vi "test-traj-generate-8-way.vi"() -> ()   [LabVIEW 2019]
uses:
  <vilib>/Rock Robotics/WPI/ThirdParty/JAS_Junk/TrajLib/TRAJECTORY.ctl
  <vilib>/Rock Robotics/WPI/ThirdParty/JAS_Junk/TrajLib/TRAJ_STATE.ctl
  <vilib>/Rock Robotics/WPI/ThirdParty/JAS_Junk/TrajLib/POSE2D.ctl
  <vilib>/Rock Robotics/WPI/ThirdParty/JAS_Junk/TrajLib/TRANSLATION2D.ctl
  <vilib>/Rock Robotics/WPI/ThirdParty/JAS_Junk/TrajLib/ROTATION2D.ctl
  <vilib>/Rock Robotics/WPI/ThirdParty/JAS_Junk/TrajLib/UTIL_WAYPOINT.ctl
  <vilib>/Rock Robotics/WPI/ThirdParty/JAS_Junk/TrajLib/SPLINE.ctl
  <vilib>/Analysis/Matrix/Datatypes/RealMatrix.ctl
  <vilib>/Rock Robotics/WPI/ThirdParty/JAS_Junk/TrajLib/POSEwCURVATURE.ctl
  <vilib>/Rock Robotics/WPI/ThirdParty/JAS_Junk/TrajLib/TRAJ_CONFIG.ctl
  <vilib>/Rock Robotics/WPI/ThirdParty/JAS_Junk/TrajLib/TRAJ_CONSTRAINT_DIIF_DRIVE_KINEMATICS.ctl
  <vilib>/Rock Robotics/WPI/ThirdParty/JAS_Junk/TrajLib/DIFF_DRIVE_KINEMATICS.ctl
  <vilib>/Rock Robotics/WPI/ThirdParty/JAS_Junk/TrajLib/TRAJ_CONSTRAINT_CENTRIPETAL_ACCEL.ctl
  <vilib>/Rock Robotics/WPI/ThirdParty/JAS_Junk/TrajLib/TRAJ_CONSTRAINT_SWERVE_DRIVE_KINEMATICS.ctl
  <vilib>/Rock Robotics/WPI/ThirdParty/JAS_Junk/TrajLib/SWERVE_DRIVE_KINEMATICS.ctl
  <vilib>/Rock Robotics/WPI/ThirdParty/JAS_Junk/TrajLib/TRAJ_CONSTRAINT_DIIF_DRIVE_VOLTAGE.ctl
  <vilib>/Rock Robotics/WPI/ThirdParty/JAS_Junk/TrajLib/SIMPLE_MOTOR_FF.ctl
  <vilib>/Rock Robotics/WPI/ThirdParty/JAS_Junk/TrajLib/TRAJ_CONSTRAINT_MECA_DRIVE_KINEMATICS.ctl
  <vilib>/Rock Robotics/WPI/ThirdParty/JAS_Junk/TrajLib/MECA_DRIVE_KINEMATICS.ctl
  <vilib>/Rock Robotics/WPI/ThirdParty/JAS_Junk/TrajLib/UTIL_WEIGHTED_WAYPOINT.ctl
  <vilib>/Rock Robotics/SystemInterfaces/NetworkCommunication/NetComm_UsageReport_report.vi
  <vilib>/Rock Robotics/WPI/ThirdParty/JAS_Junk/TrajLib/DiffDriveKinematicsConstraint_New.vi
  <vilib>/Rock Robotics/WPI/ThirdParty/JAS_Junk/TrajLib/CentripetalAccelConstraint_New.vi
  <vilib>/Rock Robotics/WPI/ThirdParty/JAS_Junk/TrajLib/Rotation_CreateAngle.vi
  <vilib>/Rock Robotics/WPI/ThirdParty/JAS_Junk/TrajLib/Translation_Create.vi
  <vilib>/Rock Robotics/WPI/ThirdParty/JAS_Junk/TrajLib/Util_LibraryGlobals.vi
  <vilib>/Rock Robotics/WPI/ThirdParty/JAS_Junk/TrajLib/Trajectory_Library.lvlib
  <vilib>/Analysis/Matrix/NI_Matrix.lvlib
panel:
  in  "Tab Control":T1(tab)
  in  "Interior WAYPOINTS":T2[](array[typedef])=[{"X"=1.5, "Y"=1.5}, {"X"=0.0, "Y"=0.0}, {"X"=-1.5, "Y"=-1.5}, {"X"=-3.0, "Y"=0.0}, {"X"=-1.5, "Y"=1.5}, {"X"=0.0, "Y"=0.0}, {"X"=1.5, "Y"=-1.5}] {"Y" format="%14.3f"; "X" format="%14.3f"}
  in  "Initial_Position":T3={"X"=3.0, "Y"=0.0, "ANGLE"=1.571} {"ANGLE" format="%13.3f"; "Y" format="%13.3f"; "X" format="%13.3f"}
  in  "Ending_Position":T3={"X"=3.0, "Y"=0.0, "ANGLE"=1.571} {"ANGLE" format="%13.3f"; "Y" format="%13.3f"; "X" format="%13.3f"}
  out "splines":T4[](array[typedef])
  out "ArrayPoseWithCurvature":T6[](array[typedef]) {"POSE"."ROTATION"."SIN" format="%13.4f"; "POSE"."ROTATION"."COS" format="%13.4f"; "POSE"."ROTATION"."VALUE" format="%13.4f"; "POSE"."TRANSLATION"."Y" format="%14.3f"; "POSE"."TRANSLATION"."X" format="%14.3f"}
  out "PoseCSize":i32
  out "error out 2":errorcluster
  in  "MaxVelocity":dbl=2.0 format="%17.4f"
  in  "MaxAcceleration":dbl=1.3 format="%17.4f"
  in  "TrackWidth_Meters":dbl=0.66 format="%20.4f"
  in  "Max Cent Accel":dbl=1.0 format="%20.4f"
  out "outTRAJECTORY_CONFIG":T9={"MaxVelocity"=0.0, "Max Acceleration"=0.0, "StartVelocity"=0.0, "End Velocity"=0.0, "Reversed"=FALSE, "DiffDrKineConstntDefined"=FALSE, "CentAcellConstntDefined"=FALSE, "DiffDrVoltConstntDefined"=FALSE, "DIFF_DRIVE_KINE_CONSTRAINT"={"Max Speed (M/S)"=0.0, "DIFF_DRIVE_KINEMATICS"={"TrackWidth_Meters"=0.0}}, "CENTRIPETAL_ACCEL_CONSTRAINT"={"Max Cent Accel"=0.0}, "SwerveDrKineConstntDefined"=FALSE, "SWERVE_DRIVE_KINE_CONSTRAINT"={"Max Speed (M/S)"=0.0, "SwerveKinematics"={"NumModules"=0, "InverseKinematics"=[], "ForwardKinematics"=[], "Modules"=[], "PrevCoR"={"X"=0.0, "Y"=0.0}}}, "DIFF_DRIVE_VOLTAGE_CONSTRAINT"={"Max Voltage"=0.0, "DIFF_DRIVE_KINEMATICS"={"TrackWidth_Meters"=0.0}, "SIMPLE_MOTOR_FF"={"Ks"=0.0, "Kv"=0.0, "Ka"=0.0}}, "MECANUM_DRIVE_KINE_CONSTRAINT"={"Max Speed (M/S)"=0.0, "MECA_DRIVE_KINEMATICS"={"FrontLeft"={"X"=0.0, "Y"=0.0}, "FrontRight"={"X"=0.0, "Y"=0.0}, "RearLeft"={"X"=0.0, "Y"=0.0}, "RearRight"={"X"=0.0, "Y"=0.0}, "InverseKinematics"=[[0.0, 1.0, -1.0, 0.0], [0.0, 1.0, 1.0, 0.0], [0.0, 1.0, 1.0, 0.0], [0.0, 1.0, -1.0, 0.0]], "ForwardKinematics"=[[0.0, 1.0, -1.0, 0.0], [0.0, 1.0, 1.0, 0.0], [0.0, 1.0, 1.0, 0.0], [0.0, 1.0, -1.0, 0.0]], "PrevCoR"={"X"=0.0, "Y"=0.0}}}, "MecanumDrKineConstntDefined"=FALSE} {"MECANUM_DRIVE_KINE_CONSTRAINT"."MECA_DRIVE_KINEMATICS"."PrevCoR"."Y" format="%14.3f"; "MECANUM_DRIVE_KINE_CONSTRAINT"."MECA_DRIVE_KINEMATICS"."PrevCoR"."X" format="%14.3f"; "MECANUM_DRIVE_KINE_CONSTRAINT"."MECA_DRIVE_KINEMATICS"."RearRight"."Y" format="%14.3f"; "MECANUM_DRIVE_KINE_CONSTRAINT"."MECA_DRIVE_KINEMATICS"."RearRight"."X" format="%14.3f"; "MECANUM_DRIVE_KINE_CONSTRAINT"."MECA_DRIVE_KINEMATICS"."RearLeft"."Y" format="%14.3f"; "MECANUM_DRIVE_KINE_CONSTRAINT"."MECA_DRIVE_KINEMATICS"."RearLeft"."X" format="%14.3f"; "MECANUM_DRIVE_KINE_CONSTRAINT"."MECA_DRIVE_KINEMATICS"."FrontRight"."Y" format="%14.3f"; "MECANUM_DRIVE_KINE_CONSTRAINT"."MECA_DRIVE_KINEMATICS"."FrontRight"."X" format="%14.3f"; "MECANUM_DRIVE_KINE_CONSTRAINT"."MECA_DRIVE_KINEMATICS"."FrontLeft"."Y" format="%14.3f"; "MECANUM_DRIVE_KINE_CONSTRAINT"."MECA_DRIVE_KINEMATICS"."FrontLeft"."X" format="%14.3f"; "MECANUM_DRIVE_KINE_CONSTRAINT"."Max Speed (M/S)" format="%20.4f"; "DIFF_DRIVE_VOLTAGE_CONSTRAINT"."SIMPLE_MOTOR_FF"."Ka" format="%13.4f"; "DIFF_DRIVE_VOLTAGE_CONSTRAINT"."SIMPLE_MOTOR_FF"."Kv" format="%13.4f"; "DIFF_DRIVE_VOLTAGE_CONSTRAINT"."SIMPLE_MOTOR_FF"."Ks" format="%13.4f"; "DIFF_DRIVE_VOLTAGE_CONSTRAINT"."DIFF_DRIVE_KINEMATICS"."TrackWidth_Meters" format="%20.4f"; "DIFF_DRIVE_VOLTAGE_CONSTRAINT"."Max Voltage" format="%20.4f"; "SWERVE_DRIVE_KINE_CONSTRAINT"."SwerveKinematics"."PrevCoR"."Y" format="%14.3f"; "SWERVE_DRIVE_KINE_CONSTRAINT"."SwerveKinematics"."PrevCoR"."X" format="%14.3f"; "SWERVE_DRIVE_KINE_CONSTRAINT"."SwerveKinematics"."Modules"."Y" format="%14.3f"; "SWERVE_DRIVE_KINE_CONSTRAINT"."SwerveKinematics"."Modules"."X" format="%14.3f"; "SWERVE_DRIVE_KINE_CONSTRAINT"."Max Speed (M/S)" format="%20.4f"; "CENTRIPETAL_ACCEL_CONSTRAINT"."Max Cent Accel" format="%20.4f"; "DIFF_DRIVE_KINE_CONSTRAINT"."DIFF_DRIVE_KINEMATICS"."TrackWidth_Meters" format="%20.4f"; "DIFF_DRIVE_KINE_CONSTRAINT"."Max Speed (M/S)" format="%20.4f"; "End Velocity" format="%20.4f"; "StartVelocity" format="%20.4f"; "Max Acceleration" format="%20.4f"; "MaxVelocity" format="%20.4f"}
  out "TRAJECTORY":T19 {"States"."POSE"."ROTATION"."SIN" format="%13.4f"; "States"."POSE"."ROTATION"."COS" format="%13.4f"; "States"."POSE"."ROTATION"."VALUE" format="%13.4f"; "States"."POSE"."TRANSLATION"."Y" format="%14.3f"; "States"."POSE"."TRANSLATION"."X" format="%14.3f"; "TotalTImeSecs" format="%20.3f"}
  out "size(s)":i32
  out "error out":errorcluster
  out "read Traj":errorcluster
  out "readTRAJECTORY":T19 {"States"."POSE"."ROTATION"."SIN" format="%13.4f"; "States"."POSE"."ROTATION"."COS" format="%13.4f"; "States"."POSE"."ROTATION"."VALUE" format="%13.4f"; "States"."POSE"."TRANSLATION"."Y" format="%14.3f"; "States"."POSE"."TRANSLATION"."X" format="%14.3f"; "TotalTImeSecs" format="%20.3f"}
  out "size(s) 2":i32
  out "file write error":errorcluster
  out "appended path":path
  out "XY Graph":cluster{dbl[], dbl[]}(graph)
  out "Position":cluster{dbl[], dbl[]}(graph)
  out "Time":dbl
  in  "STEP":bool
  out "XY Graph 2":cluster{dbl[], dbl[]}(graph)
  out "TimeSeconds":dbl
  out "OutputTRAJ_STATE":T20={"TimeSeconds"=0.0, "Velocity"=0.0, "Acceleration"=0.0, "POSE"={"TRANSLATION"={"X"=0.0, "Y"=0.0}, "ROTATION"={"VALUE"=0.0, "COS"=1.0, "SIN"=0.0}}, "Curvature"=0.0} {"POSE"."ROTATION"."SIN" format="%13.4f"; "POSE"."ROTATION"."COS" format="%13.4f"; "POSE"."ROTATION"."VALUE" format="%13.4f"; "POSE"."TRANSLATION"."Y" format="%14.3f"; "POSE"."TRANSLATION"."X" format="%14.3f"}
  in  "CONT":bool
  out "Done":bool
  # "ARRAY OF OTHER\nCONSTRAINTS \nGOES HERE.."
  # "Single step\nthrough \ntrajectory"
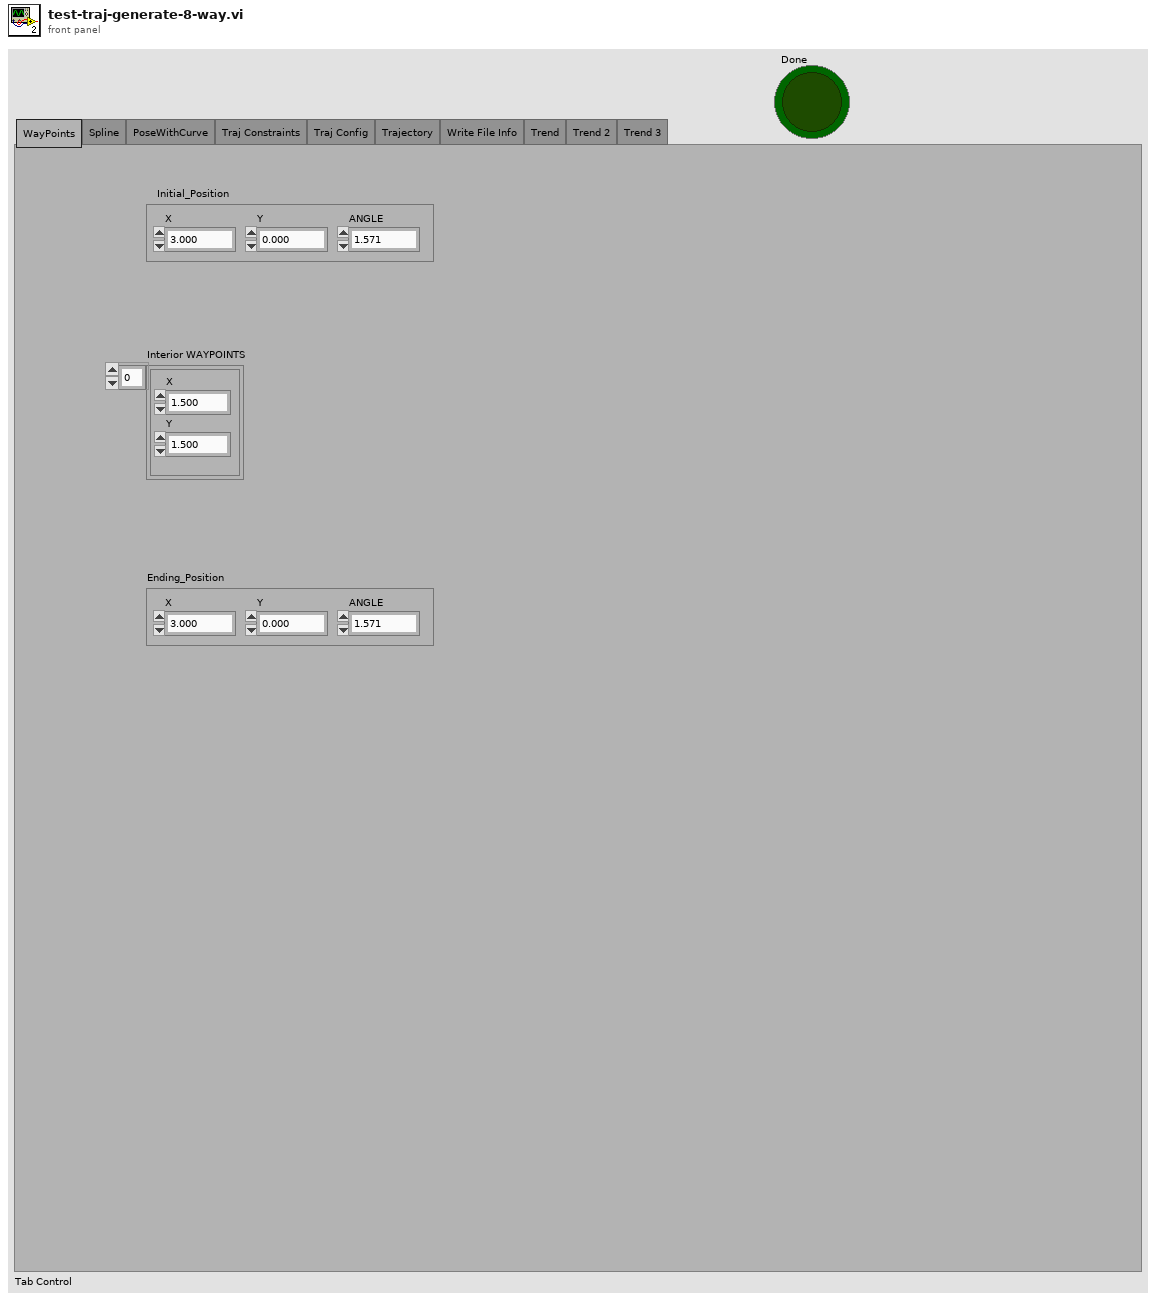
[diagram p1: front panel]
types:
  T1 = enum32{"WayPoints", "Spline", "PoseWithCurve", "Traj Constraints", "Traj Config", "Trajectory", "Write File Info", "Trend", "Trend 2", "Trend 3"}
  T2 = typedef "Trajectory_Library.lvlib/TRANSLATION2D.ctl" = cluster{"X":dbl, "Y":dbl}
  T3 = typedef "Trajectory_Library.lvlib/UTIL_WAYPOINT.ctl" = cluster{"X":dbl, "Y":dbl, "ANGLE":dbl}
  T4 = typedef "Trajectory_Library.lvlib/SPLINE.ctl" = cluster{"Degree":i32, "Coefficients":T5}
  T5 = typedef "NI_Matrix.lvlib/RealMatrix.ctl" = dbl[][]
  T6 = typedef "Trajectory_Library.lvlib/POSEwCURVATURE.ctl" = cluster{"CURVATURE":dbl, "POSE":T7}
  T7 = typedef "Trajectory_Library.lvlib/POSE2D.ctl" = cluster{"TRANSLATION":T2, "ROTATION":T8}
  T8 = typedef "Trajectory_Library.lvlib/ROTATION2D.ctl" = cluster{"VALUE":dbl, "COS":dbl, "SIN":dbl}
  T9 = typedef "Trajectory_Library.lvlib/TRAJ_CONFIG.ctl" = cluster{"MaxVelocity":dbl, "Max Acceleration":dbl, "StartVelocity":dbl, "End Velocity":dbl, "Reversed":bool, "DiffDrKineConstntDefined":bool, "CentAcellConstntDefined":bool, "DiffDrVoltConstntDefined":bool, "DIFF_DRIVE_KINE_CONSTRAINT":T10, "CENTRIPETAL_ACCEL_CONSTRAINT":T12, "SwerveDrKineConstntDefined":bool, "SWERVE_DRIVE_KINE_CONSTRAINT":T13, "DIFF_DRIVE_VOLTAGE_CONSTRAINT":T15, "MECANUM_DRIVE_KINE_CONSTRAINT":T17, "MecanumDrKineConstntDefined":bool}
  T10 = typedef "Trajectory_Library.lvlib/TRAJ_CONSTRAINT_DIIF_DRIVE_KINEMATICS.ctl" = cluster{"Max Speed (M/S)":dbl, "DIFF_DRIVE_KINEMATICS":T11}
  T11 = typedef "Trajectory_Library.lvlib/DIFF_DRIVE_KINEMATICS.ctl" = cluster{"TrackWidth_Meters":dbl}
  T12 = typedef "Trajectory_Library.lvlib/TRAJ_CONSTRAINT_CENTRIPETAL_ACCEL.ctl" = cluster{"Max Cent Accel":dbl}
  T13 = typedef "Trajectory_Library.lvlib/TRAJ_CONSTRAINT_SWERVE_DRIVE_KINEMATICS.ctl" = cluster{"Max Speed (M/S)":dbl, "SwerveKinematics":T14}
  T14 = typedef "Trajectory_Library.lvlib/SWERVE_DRIVE_KINEMATICS.ctl" = cluster{"NumModules":i32, "InverseKinematics":T5, "ForwardKinematics":T5, "Modules":T2[], "PrevCoR":T2}
  T15 = typedef "Trajectory_Library.lvlib/TRAJ_CONSTRAINT_DIIF_DRIVE_VOLTAGE.ctl" = cluster{"Max Voltage":dbl, "DIFF_DRIVE_KINEMATICS":T11, "SIMPLE_MOTOR_FF":T16}
  T16 = typedef "Trajectory_Library.lvlib/SIMPLE_MOTOR_FF.ctl" = cluster{"Ks":dbl, "Kv":dbl, "Ka":dbl}
  T17 = typedef "Trajectory_Library.lvlib/TRAJ_CONSTRAINT_MECA_DRIVE_KINEMATICS.ctl" = cluster{"Max Speed (M/S)":dbl, "MECA_DRIVE_KINEMATICS":T18}
  T18 = typedef "Trajectory_Library.lvlib/MECA_DRIVE_KINEMATICS.ctl" = cluster{"FrontLeft":T2, "FrontRight":T2, "RearLeft":T2, "RearRight":T2, "InverseKinematics":T5, "ForwardKinematics":T5, "PrevCoR":T2}
  T19 = typedef "Trajectory_Library.lvlib/TRAJECTORY.ctl" = cluster{"TotalTImeSecs":dbl, "States":T20[]}
  T20 = typedef "Trajectory_Library.lvlib/TRAJ_STATE.ctl" = cluster{"TimeSeconds":dbl, "Velocity":dbl, "Acceleration":dbl, "POSE":T7, "Curvature":dbl}
  T21 = typedef "Trajectory_Library.lvlib/UTIL_WEIGHTED_WAYPOINT.ctl" = cluster{"X":dbl, "Y":dbl, "ANGLE":dbl, "WEIGHT":dbl}
  T22 = typedef "Trajectory_Library.lvlib/SPLINE_CTRL_VECTOR.ctl" = cluster{"Xs":dbl[], "Ys":dbl[]}
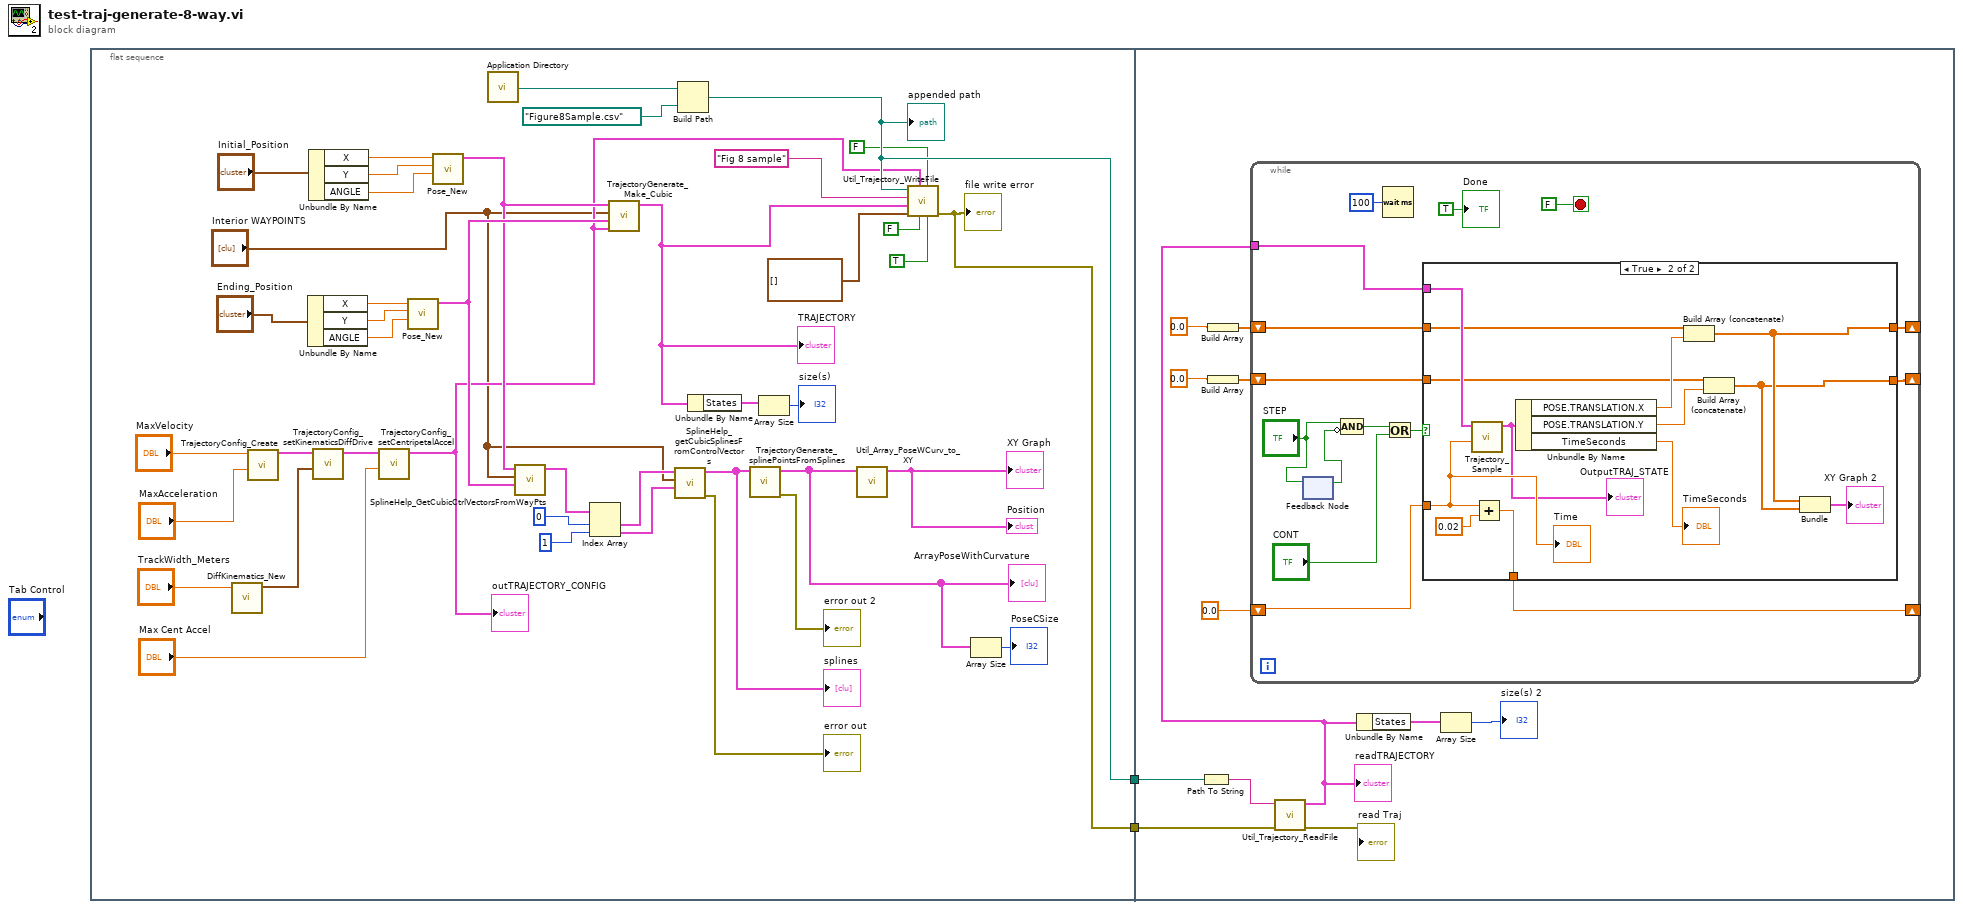
[diagram p0: block diagram]
diagram:
  n1 = flat-sequence {
    tunnel: [w11] -> w2
    tunnel: [w3] -> w1
    tunnel: w2 -> [w49]
    tunnel: w1 -> [w45]
    frame #0 {
      n2 = call <vilib>:"DiffKinematics_New.vi"("TrackWidth_Meters"="TrackWidth_Meters") -> ("DIFF_DRIVE_KINEMATICS"=w16:T11)  [unwired: 10 in]
      n3 = call <vilib>:"TrajectoryConfig_Create.vi"("MaxAcceleration"="MaxAcceleration", "MaxVelocity"="MaxVelocity") -> ("TRAJECTORY_CONFIG"=w18:T9)  [unwired: 9 in]
      n4 = Unbundle By Name("Ending_Position") -> ("X"=w40:dbl, "Y"=w39:dbl, "ANGLE"=w38:dbl)
      n5 = Unbundle By Name("Initial_Position") -> ("X"=w43:dbl, "Y"=w42:dbl, "ANGLE"=w41:dbl)
      n6 = call <vilib>:"TrajectoryConfig_setKinematicsDiffDrive.vi"("DIFF_DRIVE_KINEMATICS"=w16, "inTRAJECTORY_CONFIG"=w18) -> ("outTRAJECTORY_CONFIG"=w15:T9)  [unwired: 9 in]
      n7 = call <vilib>:"TrajectoryConfig_setCentripetalAccel.vi"("Max Cent Accel"="Max Cent Accel", "inTRAJECTORY_CONFIG"=w15) -> ("outTRAJECTORY_CONFIG"=w10:T9)  [unwired: 9 in]
      "outTRAJECTORY_CONFIG" <- w10
      n8 = call <vilib>:"Pose_New.vi"("Heading"=w38, "Y"=w39, "X"=w40) -> ("out POSe"=w36:T7)  [unwired: 8 in]
      n9 = call <vilib>:"Pose_New.vi"("Heading"=w41, "Y"=w42, "X"=w43) -> ("out POSe"=w35:T7)  [unwired: 8 in]
      n10 = call <vilib>:"Application Directory.vi"() -> ("Application Directory"=w12:path)
      n11 = call <vilib>:"SplineHelp_GetCubicCtrlVectorsFromWayPts.vi"("Enging POSE"=w36, "Interior WAYPOINTS"="Interior WAYPOINTS", "Starting POSE"=w35) -> ("SplineControlVectors"=w25:T22[])  [unwired: 8 in]
      n12 = Index Array(array=w25, index #1=0 ("index"), index #2=1 ("index")) -> (element #1=w24:T22, element #2=w23:T22)
      n13 = call <vilib>:"TrajectoryGenerate_Make_Cubic.vi"("traj_config"=w10, "Enging POSE"=w36, "Interior WAYPOINTS"="Interior WAYPOINTS", "Starting POSE"=w35) -> ("TRAJECTORY"=w22:T19)  [unwired: 6 in, 1 out]
      "TRAJECTORY" <- w22
      n14 = call <vilib>:"SplineHelp_getCubicSplinesFromControlVectors.vi"("endCtrlVector"=w23, "InternalWaypoints"="Interior WAYPOINTS", "startCtrlVector"=w24) -> ("error out"=→"error out":errorcluster, "splines"=w33:T4[])  [unwired: 3 in, 4 out]
      "splines" <- w33
      n15 = Build Path(base path=w12, name or relative path=path "Figure8Sample.csv" ("Trajectory File Name")) -> (appended path=w11:path)
      "appended path" <- w11
      n16 = Unbundle By Name(w22) -> ("States"=w31:T20[])
      n17 = call <vilib>:"TrajectoryGenerate_splinePointsFromSplines.vi"("inputSPLINE"=w33) -> ("error out"=→"error out 2":errorcluster, "ArrayPoseWithCurvature"=w8:T6[])  [unwired: 9 in]
      "ArrayPoseWithCurvature" <- w8
      n18 = Array Size(array=w31) -> (size(s)=→"size(s)":i32)
      n19 = call <vilib>:"Util_Array_PoseWCurv_to_XY.vi"("inArrayPoseWCurve"=w8) -> ("outArrayXY"=→"XY Graph" →"Position":cluster{dbl[], dbl[]})  [unwired: 10 in]
      n20 = call <vilib>:"Util_Trajectory_WriteFile.vi"("Trajectory is Cubic"=TRUE, "UseWeights"=FALSE, "Trajectory Is Relative"=FALSE, "TRAJECTORY_CONFIG"=w10, "UtilityWayPoints"=T21[] [], "TRAJECTORY"=w22, "Comment"="Fig 8 sample", "Trajectory File Name"=w11) -> ("error out"=w3:errorcluster)  [unwired: 3 in]
      "file write error" <- w3
      n21 = Array Size(array=w8) -> (size(s)=→"PoseCSize":i32)
    }
    frame #1 {
      n22 = Path To String(path=w49) -> (string=w50:string)
      n23 = Build Array(0.0) -> (w53:dbl[])
      n24 = Build Array(0.0) -> (w52:dbl[])
      n25 = call <vilib>:"Util_Trajectory_ReadFile.vi"("error in (no error)"=w45, "FileName"=w50) -> ("error out"=→"read Traj":errorcluster, "outTRAJECTORY"=w46:T19)  [unwired: 8 in]
      "readTRAJECTORY" <- w46
      n26 = while {
        shift-right: [w67] -> _
        shift-left: 0.0 -> [w68]
        tunnel: w46 -> [w64]
        shift-right: [w63] -> _
        shift-left: w53 -> [w66]
        shift-right: [w62] -> _
        shift-left: w52 -> [w65]
        stop <- FALSE stop-if-true
        n27 = feedback-in #1("STEP") -> ()
        n28 = feedback #1() -> (w60:bool)  [unwired: 1 in]
        n29 = Compound Arithmetic op=AND("STEP", invert w60) -> (w58:bool)
        n30 = Wait (ms)(milliseconds to wait=u32 100) -> ()  [unwired: 1 out]
        n31 = Or(x=w58, y="CONT") -> (x .or. y?=w59:bool)
        n32 = case shown="True" w59 {
          tunnel: w68 -> [w74 w85]
          tunnel: [w74 w87] -> w67
          tunnel: w66 -> [w73 w81]
          tunnel: w65 -> [w72 w79]
          tunnel: w64 -> [_ w84]
          tunnel: [w73 w76] -> w63
          tunnel: [w72 w75] -> w62
          frame False {
          }
          frame True {
            n33 = call <vilib>:"Trajectory_Sample.vi"("Time"=w85, "InputTRAJECTORY"=w84) -> ("OutputTRAJ_STATE"=w83:T20)  [unwired: 9 in]
            "OutputTRAJ_STATE" <- w83
            n34 = Add(x=w85, y=0.02) -> (x+y=w87:dbl)
            n35 = Unbundle By Name(w83) -> ("POSE.TRANSLATION.X"=w80:dbl, "POSE.TRANSLATION.Y"=w78:dbl, "TimeSeconds"=→"TimeSeconds":dbl)
            n36 = Build Array (concatenate)(w81, w80) -> (w76:dbl[])
            n37 = Build Array (concatenate)(w79, w78) -> (w75:dbl[])
            n38 = Bundle(w76, w75) -> (→"XY Graph 2":cluster{dbl[], dbl[]})  [unwired: 1 in]
            "Time" <- w85
          }
        }
        "Done" <- TRUE ("Done")
      }
      n39 = Unbundle By Name(w46) -> ("States"=w48:T20[])
      n40 = Array Size(array=w48) -> (size(s)=→"size(s) 2":i32)
    }
  }
